vi "DAQ Finite Read Servo Errors.vi"(5 "samples per channel":i32=1000, 7 "rate":dbl=1000.0 caption="Samples per Second" format="%0.2f", 8 "error in":errorcluster, 10 "task/channels in":refnum<k21>, 11 "Action":T1) -> (0 "error out":errorcluster, 2 "Average":dbl[](array[numeric]))   [LabVIEW 2009]
uses:
  Test Utilities/DAQ Read Actions.ctl
  <vilib>/DAQmx/configure/timing.llb/DAQmx Timing (Sample Clock).vi
  <vilib>/DAQmx/read.llb/DAQmx Read (Analog 2D DBL NChan NSamp).vi
panel:
  out "Data":dbl[][](array[numeric]) format="%0.2f"
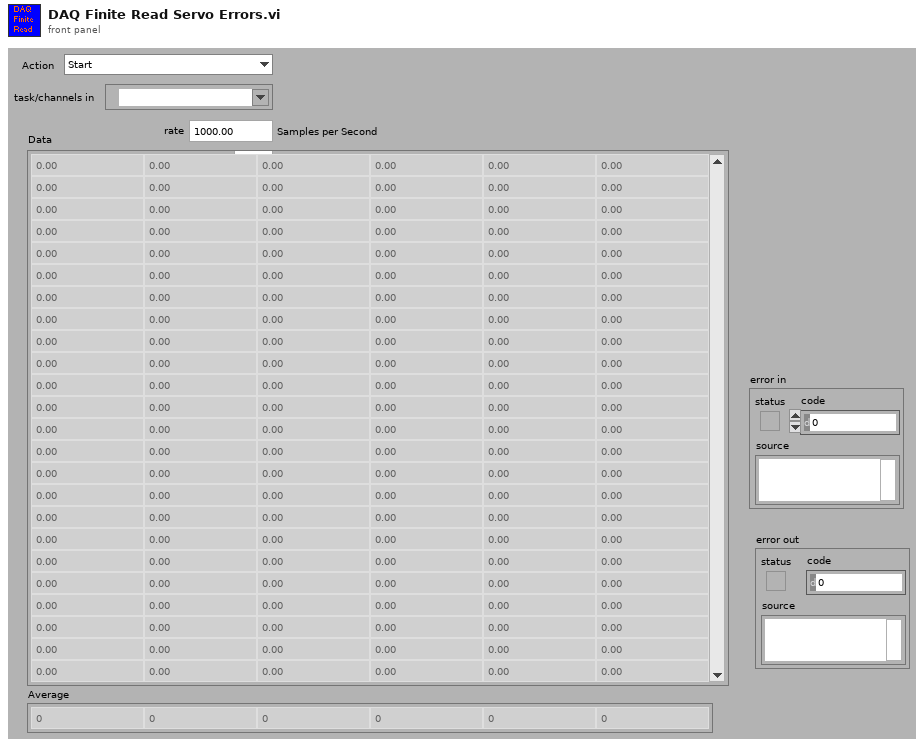
[diagram p1: front panel]
types:
  T1 = typedef "DAQ Read Actions.ctl" = enum16{"Start", "Read", "Stop"}
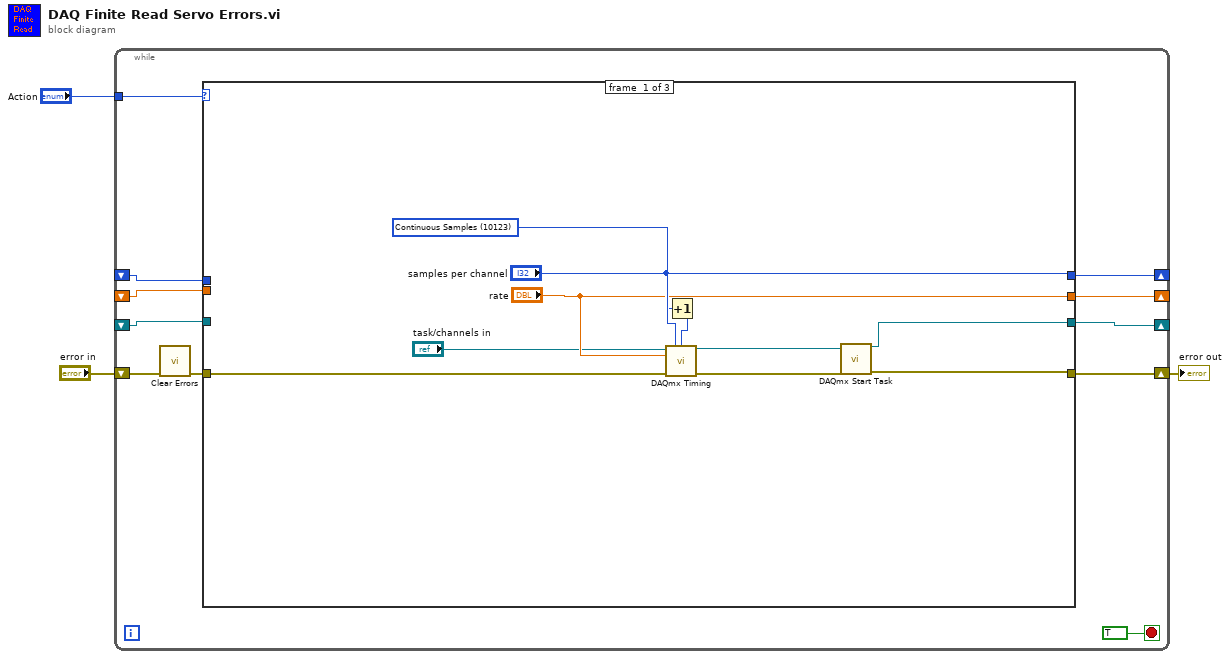
[diagram p0: block diagram]
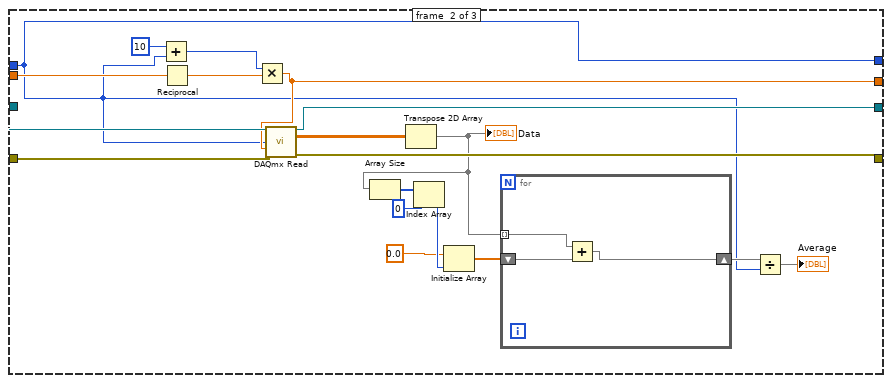
[diagram p2: hidden frame]
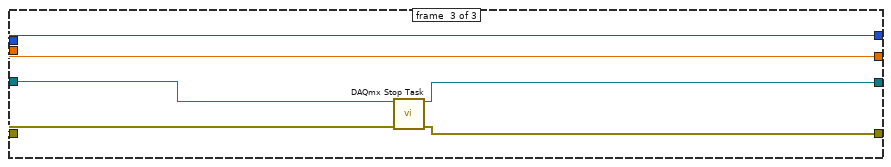
[diagram p3: hidden frame]
diagram:
  n1 = while {
    tunnel: "Action" -> [w13]
    shift-right: [w4] -> w2
    shift-left: "error in" -> [w12]
    shift-right: [w11] -> _
    shift-left: _ -> [w10]
    shift-right: [w8] -> _
    shift-left: _ -> [w6]
    shift-right: [w9] -> _
    shift-left: _ -> [w7]
    stop <- TRUE stop-if-true
    n2 = call <vilib>:"Clear Errors.vi"("error in (no error)"=w12) -> ("error out"=w5:errorcluster)  [unwired: 6 out]
    n3 = case shown="\"Read\"" w13 {
      tunnel: [w16 w42 w49] -> w4
      tunnel: w5 -> [w20 w38 w51]
      tunnel: [w17 w43 w50] -> w11
      tunnel: w10 -> [_ w37 w52]
      tunnel: ["samples per channel" w25 w47] -> w9
      tunnel: ["rate" w27 w48] -> w8
      tunnel: w7 -> [_ w25 w47]
      tunnel: w6 -> [_ w41 w48]
      frame #0 {
        w24 = 10123 items=["Finite Samples"=10178, "Continuous Samples"=10123, "Hardware Timed Single Point"=12522] ("sample mode")
        n4 = Increment(x="samples per channel") -> (x+1=w15:i32)
        n5 = call-poly <vilib>:"DAQmx Timing.vi"("task/channels in"="task/channels in", "sample mode"=w24, "samples per channel"=w15, "rate"="rate", "error in"=w20) -> ("task out"=w18:refnum<k21>, "error out"=w19:errorcluster)  [unwired: 2 in, 7 out]
        n6 = call <vilib>:"DAQmx Start Task.vi"("task/channels in"=w18, "error in"=w19) -> ("task out"=w17:refnum<k21>, "error out"=w16:errorcluster)  [unwired: 12 out]
      }
      frame #1 {
        n7 = Add(x=10, y=w25) -> (x+y=w36:i32)
        n8 = Reciprocal(x=w41) -> (1/x=w26:dbl)
        n9 = Multiply(x=w36, y=w26) -> (x*y=w27:dbl)
        n10 = call-poly <vilib>:"DAQmx Read.vi"("task/channels in"=w37, "number of samples per channel"=w25, "timeout"=w27, "error in"=w38) -> ("task out"=w43:refnum<k21>, "data"=w39:dbl[][], "error out"=w42:errorcluster)  [unwired: 9 out]
        n11 = Transpose 2D Array(2D array=w39) -> (transposed array=w33:dbl[][])
        "Data" <- w33
        n12 = Array Size(array=w33) -> (size(s)=w32:i32[])
        n13 = Index Array(array=w32, index=0) -> (element=w29:i32)
        n14 = Initialize Array(0.0 ("element"), w29) -> (w30:dbl[])
        n15 = for {
          shift-right: [w45] -> w35
          shift-left: w30 -> [w44]
          tunnel: w33 -> [w46] mode=indexing
          n16 = Add(x=w46, y=w44) -> (x+y=w45:dbl[])
        }
        n17 = Divide(x=w35, y=w25) -> (x/y=→"Average":dbl[])
      }
      frame #2 {
        n18 = call <vilib>:"DAQmx Stop Task.vi"("task/channels in"=w52, "error in"=w51) -> ("task out"=w50:refnum<k21>, "error out"=w49:errorcluster)  [unwired: 12 out]
      }
    }
  }
  "error out" <- w2
